vi "Drive Core.vi"() -> ()   [LabVIEW 2014]
uses:
  <vilib>/Rock Robotics/WPI/DriverStation/WPI_DriverStationRobotMode2.ctl
  <vilib>/Rock Robotics/Network Tables/SD Read Boolean.vi
  Begin/Global Variables.vi
  Begin/Global Constants.vi
  Begin/Global RefNums.vi
panel:
  in  "Min Correction":dbl=0.1
  in  "Reset Encoders":bool
  out "Counts FR":i32=881
  out "Counts FL":i32=731
  out "Counts BR":i32=531
  out "Counts BL":i32=477
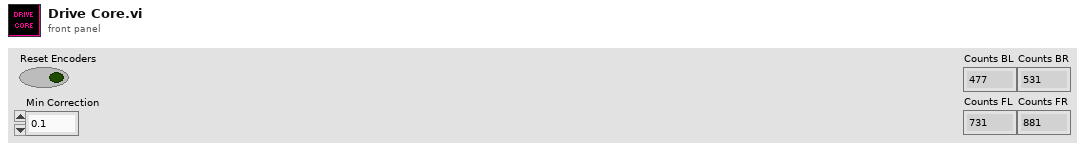
[diagram p1: front panel]
types:
  T1 = cluster{"Header P":dbl, "Header I":dbl, "Header D":dbl}
  T2 = typedef "WPI_DriverStationRobotMode2.ctl" = enum16{"Autonomous Disabled", "Autonomous Enabled", "Teleop Disabled", "Teleop Enabled", "Disconnected", "Finish", "Test Disabled", "Test Enabled", "Emergency Stopped"}
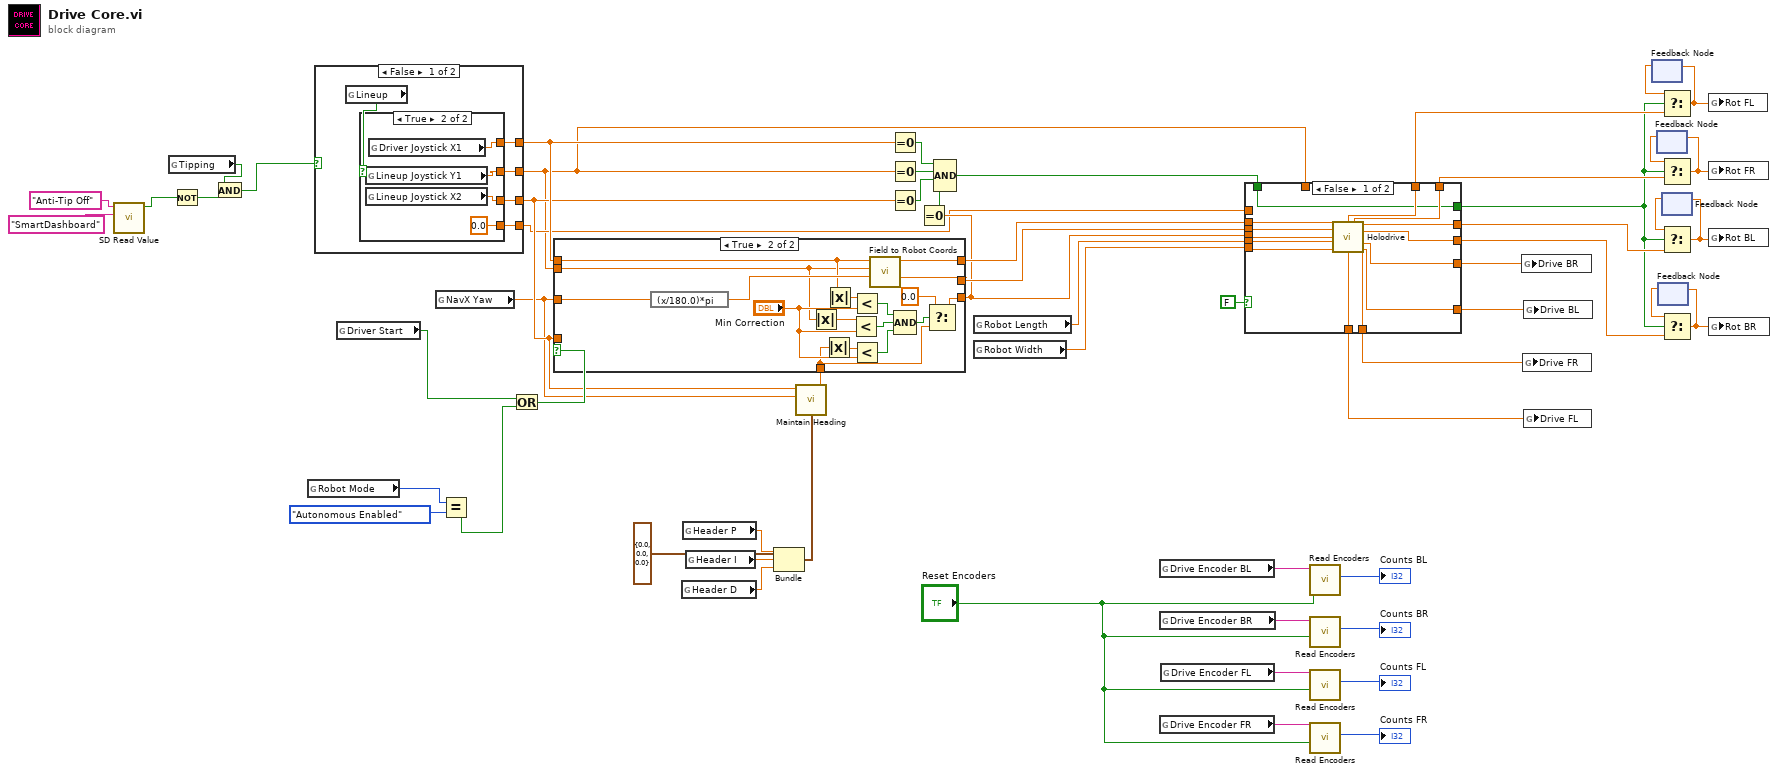
[diagram p0: block diagram]
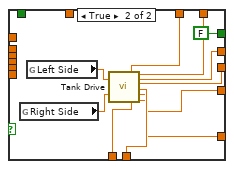
[diagram p2: hidden frame]
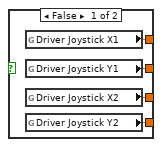
[diagram p3: hidden frame]
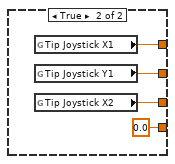
[diagram p4: hidden frame]
diagram:
  n1 = call-poly <vilib>:"SD Read Value.vi"("Table Prefix"="SmartDashboard", "Name"="Anti-Tip Off") -> ("Boolean"=w2:bool)  [unwired: 7 in, 2 out]
  n2 = global read "Global Variables.vi" "Tipping"() -> (w30:bool)
  n3 = Not(x=w2) -> (.not. x?=w1:bool)
  n4 = And(x=w30, y=w1) -> (x .and. y?=w29:bool)
  n5 = global read "Global Variables.vi" "Robot Mode"() -> (w59:T2)
  n6 = case shown="False" w29 {
    tunnel: [w64 w74] -> w23
    tunnel: [w63 w75] -> w6
    tunnel: [w62 w76] -> w58
    tunnel: [w61 0.0 ("Driver Joystick Y2")] -> w7
    frame False {
      n7 = global read "Global Variables.vi" "Lineup"() -> (w60:bool)
      n8 = case shown="True" w60 {
        tunnel: [w68 w70] -> w64
        tunnel: [w67 w71] -> w63
        tunnel: [w66 w72] -> w62
        tunnel: [w65 0.0 ("Driver Joystick Y2")] -> w61
        frame False {
          n9 = global read "Global Variables.vi" "Driver Joystick X1"() -> (w66:dbl)
          n10 = global read "Global Variables.vi" "Driver Joystick Y1"() -> (w67:dbl)
          n11 = global read "Global Variables.vi" "Driver Joystick X2"() -> (w68:dbl)
          n12 = global read "Global Variables.vi" "Driver Joystick Y2"() -> (w65:dbl)
        }
        frame True {
          n13 = global read "Global Variables.vi" "Lineup Joystick Y1"() -> (w71:dbl)
          n14 = global read "Global Variables.vi" "Lineup Joystick X2"() -> (w70:dbl)
          n15 = global read "Global Variables.vi" "Driver Joystick X1"() -> (w72:dbl)
        }
      }
    }
    frame True {
      n16 = global read "Global Variables.vi" "Tip Joystick X1"() -> (w76:dbl)
      n17 = global read "Global Variables.vi" "Tip Joystick Y1"() -> (w75:dbl)
      n18 = global read "Global Variables.vi" "Tip Joystick X2"() -> (w74:dbl)
    }
  }
  n19 = global read "Global Variables.vi" "Driver Start"() -> (w43:bool)
  n20 = global read "Global Variables.vi" "NavX Yaw"() -> (w22:dbl)
  n21 = Equal?(x=w59, y=WPI_DriverStationRobotMode2."Autonomous Enabled") -> (x = y?=w45:bool)
  n22 = Or(x=w43, y=w45) -> (x .or. y?=w44:bool)
  n23 = global read "Global Constants.vi" "Header D"() -> (w28:dbl)
  n24 = global read "Global Constants.vi" "Header P"() -> (w26:dbl)
  n25 = global read "Global Constants.vi" "Header I"() -> (w27:dbl)
  n26 = Bundle(cluster=T1 {"Header P"=0.0, "Header I"=0.0, "Header D"=0.0}, "Header P"=w26, "Header I"=w27, "Header D"=w28) -> (w24:T1)
  n27 = call "Maintain Heading.vi"("PID gains"=w24, "NavX Yaw"=w22, "Raw Driver Joystick X2"=w23) -> ("Driver Joystick X2"=w21:dbl)  [unwired: 8 in]
  n28 = case shown="True" w44 {
    tunnel: w58 -> [w79 w85]
    tunnel: w6 -> [w78 w82]
    tunnel: [w79 w93] -> w20
    tunnel: [w78 w96] -> w19
    tunnel: w23 -> [w77 _]
    tunnel: [w77 w92] -> w18
    tunnel: w22 -> [_ w94]
    tunnel: w21 -> [_ w80]
    frame False {
    }
    frame True {
      n29 = expression code="(x/180.0)*pi" ("degrees to radians")(w94) -> (w95:dbl)
      n30 = Absolute Value(x=w82) -> (abs(x)=w83:dbl)
      n31 = Absolute Value(x=w80) -> (abs(x)=w81:dbl)
      n32 = Absolute Value(x=w85) -> (abs(x)=w84:dbl)
      n33 = Less?(x=w83, y="Min Correction") -> (x < y?=w88:bool)
      n34 = Less?(x=w84, y="Min Correction") -> (x < y?=w89:bool)
      n35 = Less?(x=w81, y="Min Correction") -> (x < y?=w87:bool)
      n36 = call "Field to Robot Coords.vi"("gyro"=w95, "Joystick y"=w82, "Joystick x"=w85) -> ("robot y"=w96:dbl, "robot x"=w93:dbl)  [unwired: 7 in]
      n37 = Compound Arithmetic op=AND(w89, w88, w87) -> (w86:bool)
      n38 = Select(t=0.0, s=w86, f=w80) -> (s? t:f=w92:dbl)
    }
  }
  n39 = Equal To 0?(x=w58) -> (x = 0?=w46:bool)
  n40 = Equal To 0?(x=w6) -> (x = 0?=w47:bool)
  n41 = Equal To 0?(x=w23) -> (x = 0?=w48:bool)
  n42 = Equal To 0?(x=w18) -> (x = 0?=w42:bool)
  n43 = Compound Arithmetic op=AND(w46, w47, w48, w42) -> (w5:bool)
  n44 = global read "Global Constants.vi" "Robot Length"() -> (w17:dbl)
  n45 = global read "Global Constants.vi" "Robot Width"() -> (w16:dbl)
  n46 = global read "Global RefNums.vi" "Drive Encoder BL"() -> (w41:string)
  n47 = global read "Global RefNums.vi" "Drive Encoder BR"() -> (w40:string)
  n48 = global read "Global RefNums.vi" "Drive Encoder FR"() -> (w38:string)
  n49 = global read "Global RefNums.vi" "Drive Encoder FL"() -> (w39:string)
  n50 = case shown="False" FALSE {
    tunnel: w20 -> [w110 _]
    tunnel: w19 -> [w109 _]
    tunnel: w18 -> [w108 _]
    tunnel: w17 -> [w107 _]
    tunnel: w16 -> [w106 _]
    tunnel: [w105 w121] -> w15
    tunnel: [w104 w120] -> w14
    tunnel: [w103 w119] -> w13
    tunnel: [w102 w118] -> w12
    tunnel: [w101 w114] -> w11
    tunnel: [w100 w116] -> w10
    tunnel: [w99 w117] -> w9
    tunnel: [w98 w115] -> w8
    tunnel: w7 -> [_ _]
    tunnel: w6 -> [_ _]
    tunnel: [w97 FALSE] -> w4
    tunnel: w5 -> [w97 _]
    frame False {
      n51 = call "Holodrive.vi"("Translation X"=w110, "Translation Y"=w109, "Angular"=w108, "Robot Length"=w107, "Robot Width"=w106) -> ("FL Rot"=w105:dbl, "FR Rot"=w104:dbl, "BL Rot"=w103:dbl, "BR Rot"=w102:dbl, "BR Drive"=w101:dbl, "FL Drive"=w98:dbl, "FR Drive"=w99:dbl, "BL Drive"=w100:dbl)  [unwired: 3 in]
    }
    frame True {
      n52 = global read "Global Variables.vi" "Right Side"() -> (w112:dbl)
      n53 = global read "Global Variables.vi" "Left Side"() -> (w113:dbl)
      n54 = call "Tank Drive.vi"("Joy y1"=w113, "Joy y2"=w112) -> ("rot FL"=w121:dbl, "Drive FL"=w115:dbl, "rot FR"=w120:dbl, "rot BL"=w119:dbl, "rot BR"=w118:dbl, "Drive FR"=w117:dbl, "Drive BL"=w116:dbl, "Drive BR"=w114:dbl)  [unwired: 10 in]
    }
  }
  n55 = call "Read Encoders.vi"("Reset Encoders"="Reset Encoders", "Encoder"=w41) -> ("Counts"=→"Counts BL":i32)  [unwired: 7 in, 2 out]
  n56 = call "Read Encoders.vi"("Reset Encoders"="Reset Encoders", "Encoder"=w40) -> ("Counts"=→"Counts BR":i32)  [unwired: 7 in, 2 out]
  n57 = call "Read Encoders.vi"("Reset Encoders"="Reset Encoders", "Encoder"=w39) -> ("Counts"=→"Counts FL":i32)  [unwired: 7 in, 2 out]
  n58 = call "Read Encoders.vi"("Reset Encoders"="Reset Encoders", "Encoder"=w38) -> ("Counts"=→"Counts FR":i32)  [unwired: 7 in, 2 out]
  n59 = global write "Global Variables.vi" "Drive BR"(w11) -> ()
  n60 = global write "Global Variables.vi" "Drive FR"(w9) -> ()
  n61 = global write "Global Variables.vi" "Drive BL"(w10) -> ()
  n62 = global write "Global Variables.vi" "Drive FL"(w8) -> ()
  n63 = feedback #1() -> (w52:dbl)  [unwired: 1 in]
  n64 = feedback #2() -> (w50:dbl)  [unwired: 1 in]
  n65 = feedback #3() -> (w56:dbl)  [unwired: 1 in]
  n66 = Select(t=w52, s=w4, f=w15) -> (s? t:f=w51:dbl)
  n67 = feedback-in #1(w51) -> ()
  n68 = Select(t=w50, s=w4, f=w14) -> (s? t:f=w49:dbl)
  n69 = feedback-in #2(w49) -> ()
  n70 = feedback #4() -> (w54:dbl)  [unwired: 1 in]
  n71 = Select(t=w54, s=w4, f=w13) -> (s? t:f=w53:dbl)
  n72 = feedback-in #4(w53) -> ()
  n73 = Select(t=w56, s=w4, f=w12) -> (s? t:f=w55:dbl)
  n74 = feedback-in #3(w55) -> ()
  n75 = global write "Global Variables.vi" "Rot FL"(w51) -> ()
  n76 = global write "Global Variables.vi" "Rot FR"(w49) -> ()
  n77 = global write "Global Variables.vi" "Rot BL"(w53) -> ()
  n78 = global write "Global Variables.vi" "Rot BR"(w55) -> ()
